vi "Shutdown Linux Real-Time (2013).vi"(8 "error in (no error)":errorcluster) -> (0 "error out":errorcluster, 3 "return value":i32)   [LabVIEW 2013]
uses:
  libc-2.17.so
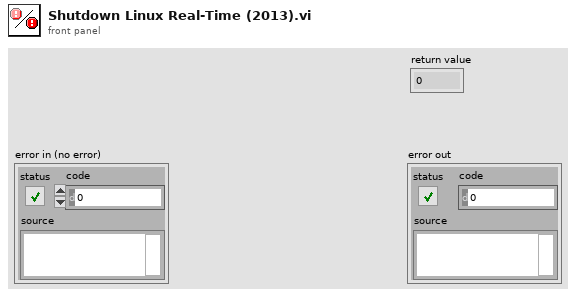
[diagram p1: front panel]
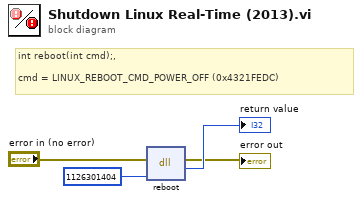
[diagram p0: block diagram]
diagram:
  # "int reboot(int cmd);, \n\ncmd = LINUX_REBOOT_CMD_POWER_OFF (0x4321FEDC)"
  n1 = dll-call lib="libc-2.17.so" fn="reboot"(error in="error in (no error)", "cmd"=1126301404 ("arg1")) -> (error out=→"error out":errorcluster, "return type"=→"return value":i32)  [unwired: 3 in, 1 out]
